vi "Create PV Data.vi"(8 "error in (no error)":errorcluster, 11 "NT Scalar in":refnum<class "NT Scalar.lvclass">) -> (0 "error out":errorcluster, 2 "PV Data out":refnum<class "PV Data.lvclass">, 3 "NT Scalar out":refnum<class "NT Scalar.lvclass">)   [LabVIEW 2020, in "PV Access.lvlib" / "PV Data.lvlib" / "NT Scalar.lvclass"]
uses:
  NT Scalar.lvclass
  PV Data/PV Data.lvclass
  NT Scalar.lvclass/NT Scalar.ctl
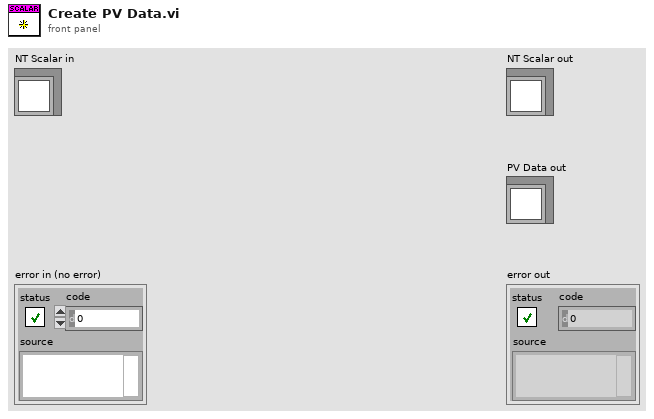
[diagram p1: front panel]
types:
  T1 = typedef "PV Access.lvlib/PV Data.lvlib/Type Code.ctl" = enum8{"Null", "Bool", "BoolA", "Int8", "Int8A", "Int16", "Int16A", "Int32", "Int32A", "Int64", "Int64A", "UInt8", "UInt8A", "UInt16", "UInt16A", "UInt32", "UInt32A", "UInt64", "UInt64A", "Float32", "Float32A", "Float64", "Float64A", "String", "StringA", "Struct", "StructA", "Union", "UnionA", "Any", "AnyA"}
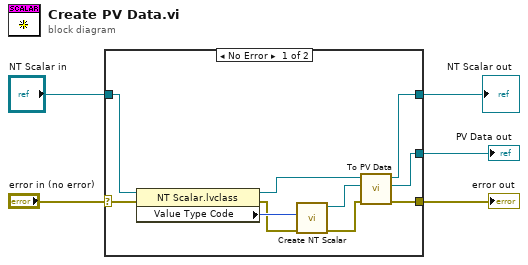
[diagram p0: block diagram]
diagram:
  n1 = case shown="No Error" "error in (no error)" {
    selector: "error in (no error)" -> [w10 w17]
    tunnel: [w14 w17] -> w3
    tunnel: [w15 w16] -> w1
    tunnel: "NT Scalar in" -> [w11 w16]
    tunnel: [w13 _] -> w2
    frame No Error {
      n2 = property class="NT Scalar.lvclass"(reference=w11, error in=w10) -> (reference out=w6:refnum<class "NT Scalar.lvclass">, error out=w8:errorcluster, "Value Type Code"=w9:T1)
      n3 = call "Create NT Scalar.vi"("error in"=w8, "type code"=w9) -> ("error out"=w12:errorcluster, "PV Data out"=w7:refnum<class "PV Data.lvclass">)  [unwired: 8 in]
      n4 = call-dynamic "To PV Data.vi"("error in"=w12, "PV data in"=w7, "Base Interface in"=w6) -> ("error out"=w14:errorcluster, "PV data out"=w13:refnum<class "PV Data.lvclass">, "Base Interface out"=w15:refnum<class "NT Scalar.lvclass">)  [unwired: 6 in]
    }
    frame Error {
    }
  }
  "error out" <- w3
  "NT Scalar out" <- w1
  "PV Data out" <- w2
